vi "getFirstDayOfQuater.vi"() -> (2 "FisrtDayofQuater":i32)   [LabVIEW 2012]
panel:
  out "date/time string":string
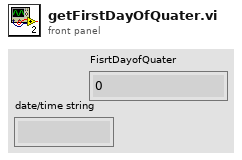
[diagram p1: front panel]
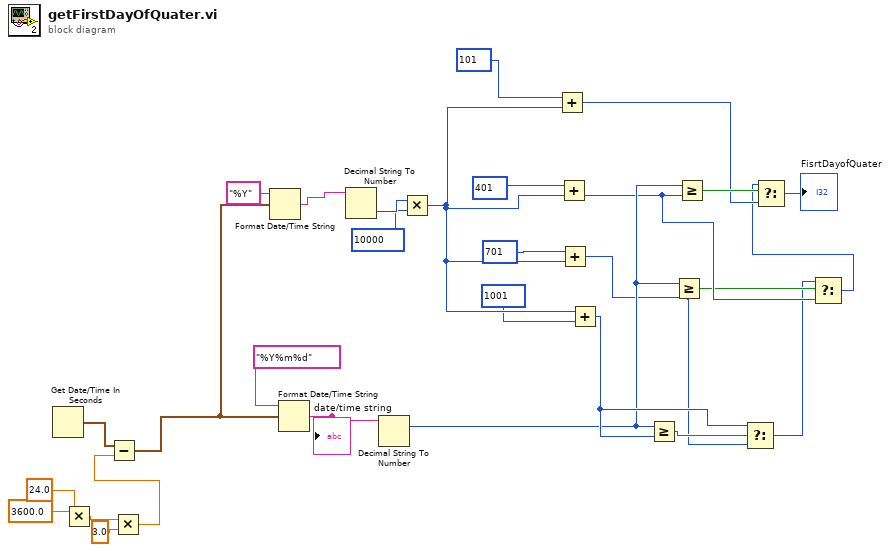
[diagram p0: block diagram]
diagram:
  n1 = Get Date/Time In Seconds() -> (seconds since 1Jan1904=w7:timestamp)
  n2 = Multiply(x=3600.0, y=24.0) -> (x*y=w3:dbl)
  n3 = Multiply(x=w3, y=3.0) -> (x*y=w1:dbl)
  n4 = Subtract(x=w7, y=w1) -> (x-y=w6:timestamp)
  n5 = Format Date/Time String(time format string (%c)="%Y", seconds (now)=w6) -> (date/time string=w27:string)  [unwired: 1 in]
  n6 = Format Date/Time String(time format string (%c)="%Y%m%d", seconds (now)=w6) -> (date/time string=w20:string)  [unwired: 1 in]
  "date/time string" <- w20
  n7 = Decimal String To Number(string=w27) -> (number=w26:i32)  [unwired: 2 in, 1 out]
  n8 = Decimal String To Number(string=w20) -> (number=w15:i32)  [unwired: 2 in, 1 out]
  n9 = Multiply(x=w26, y=10000) -> (x*y=w21:i32)
  n10 = Add(x=101, y=w21) -> (x+y=w14:i32)
  n11 = Add(x=401, y=w21) -> (x+y=w13:i32)
  n12 = Add(x=701, y=w21) -> (x+y=w10:i32)
  n13 = Add(x=w21, y=1001) -> (x+y=w17:i32)
  n14 = Greater Or Equal?(x=w15, y=w17) -> (x >= y?=w19:bool)
  n15 = Greater Or Equal?(x=w15, y=w10) -> (x >= y?=w12:bool)
  n16 = Greater Or Equal?(x=w15, y=w13) -> (x >= y?=w16:bool)
  n17 = Select(t=w17, s=w19, f=w10) -> (s? t:f=w11:i32)
  n18 = Select(t=w11, s=w12, f=w13) -> (s? t:f=w9:i32)
  n19 = Select(t=w9, s=w16, f=w14) -> (s? t:f=→"FisrtDayofQuater":i32)
